vi "dvp Vi Get Serial Number.vi"(9 "nLength":u32, 10 "SerialNumber":string, 11 "handle":u32) -> (2 "SerialNumber out":string, 3 "function return":u32(ring))   [LabVIEW 2018, in "LabViewDVPCamera.lvlib"]
doc: "LabviewDvp2Api dvpStatus dvpViGetSerialNumber(dvpHandle handle, char *SerialNumber, dvpUint32 nLength);"
uses:
  LabViewDVPCamera.lvlib
  LabViewDVPCamera/LabViewDVPCamera.dll
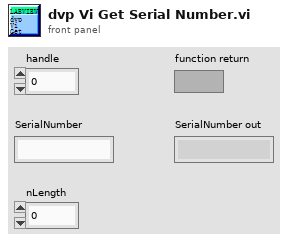
[diagram p1: front panel]
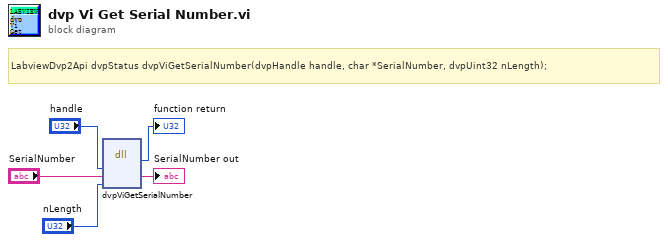
[diagram p0: block diagram]
diagram:
  # "LabviewDvp2Api dvpStatus dvpViGetSerialNumber(dvpHandle handle, char *SerialNumber, dvpUint32 nLength);"
  n1 = dll-call lib="C:/Program Files (x86)/DVP2 Labview cn 64/Sample/LabViewDVPCamera/LabViewDVPCamera.*" fn="dvpViGetSerialNumber"("handle"="handle", "SerialNumber"="SerialNumber", "nLength"="nLength") -> (→"function return":u32, "SerialNumber"=→"SerialNumber out":string)  [unwired: 5 in, 2 out]
